vi "Error Processor.vi"(8 "error in (no error)":errorcluster, 11 "Detector Manager in":refnum<class "Detector Manager.lvclass">) -> (0 "error out":errorcluster, 3 "Detector Manager out":refnum<class "Detector Manager.lvclass">)   [LabVIEW 2026, in "TALOS.lvlib" / "Detector Manager.lvlib" / "Detector Manager.lvclass"]
doc: "Use this VI to process all the error that are solvable inside this specific uService. Whatever is not possible to process, let it leave this VI and it will be processed by the Error Manager of the Distributed System."
uses:
  Detector Manager.lvclass
  Detector Manager.lvclass/Detector Manager.ctl
  Classes/Father of all Detectors/Father Of All Detectors.lvclass
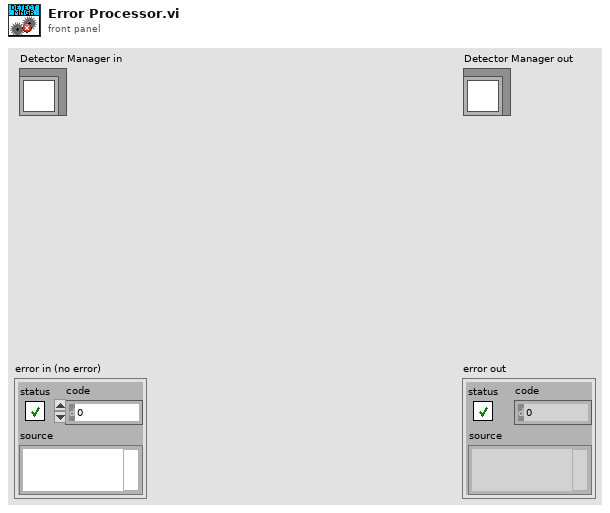
[diagram p1: front panel]
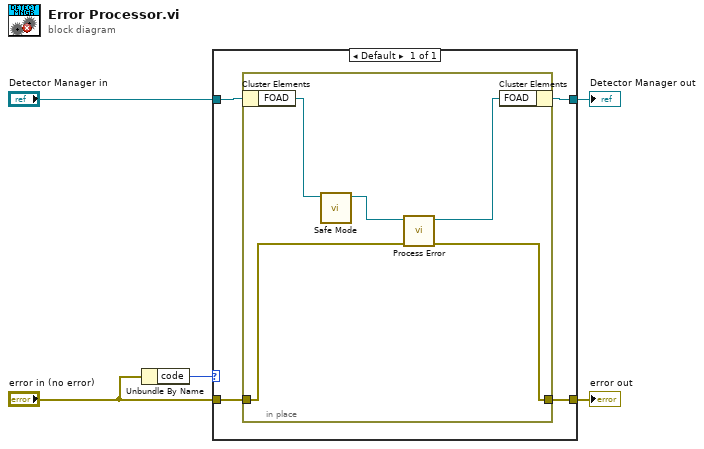
[diagram p0: block diagram]
diagram:
  n1 = Unbundle By Name("error in (no error)") -> ("code"=w3:i32)
  n2 = case shown="Default" w3 {
    tunnel: "error in (no error)" -> [w8]
    tunnel: [w7] -> w5
    tunnel: "Detector Manager in" -> [w9]
    tunnel: [w6] -> w1
    frame Default {
      n3 = in-place {
        in-place-border: w8 -> [w13]
        in-place-border: [w12] -> w7
        n4 = in-place-cluster #1(w9) -> ("FOAD"=w11:refnum<class "Father Of All Detectors.lvclass">)
        n5 = call-dynamic "Safe Mode.vi"("Father Of All Detectors in"=w11) -> ("Father Of All Detectors out"=w10:refnum<class "Father Of All Detectors.lvclass">)  [unwired: 8 in, 2 out]
        n6 = call-dynamic "Process Error.vi"("error in (no error)"=w13, "Father Of All Detectors in"=w10) -> ("error out"=w12:errorcluster, "Father Of All Detectors out"=w14:refnum<class "Father Of All Detectors.lvclass">)  [unwired: 8 in]
        n7 = in-place-cluster #1("FOAD"=w14) -> (w6:refnum<class "Detector Manager.lvclass">)
      }
    }
  }
  "error out" <- w5
  "Detector Manager out" <- w1
